vi "SetSize.vi"(9 "size":i32, 11 "PipeData in":refnum<class "StreamData.lvclass">) -> (3 "PipeData out":refnum<class "StreamData.lvclass">)   [LabVIEW 2017, in "Stream-t'WPI_EncoderType.ctl'.lvlib" / "StreamData.lvclass"]
uses:
  <extravilib>/ChannelInstances/Stream-t'WPI_EncoderType.ctl'/StreamData.lvclass
  <extravilib>/ChannelInstances/Stream-t'WPI_EncoderType.ctl'/StreamData.lvclass/StreamData.ctl
  <resource>/ChannelSupport/_ChannelSupport/PipeLogic/PipeLogic.lvclass/PipeLogic.ctl
  <resource>/ChannelSupport/_ChannelSupport/PipeLogic/PipeLogic.lvclass
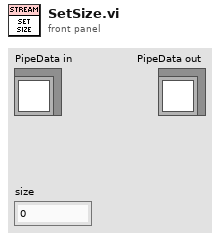
[diagram p1: front panel]
types:
  T1 = typedef "WPI_EncoderType.ctl" = enum16{"1x", "2x", "4x"}
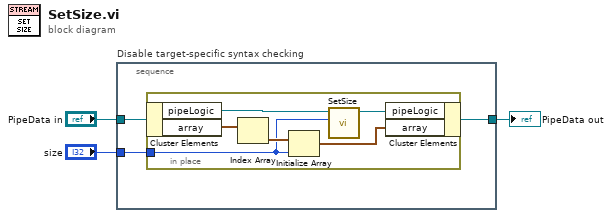
[diagram p0: block diagram]
diagram:
  n1 = stacked-sequence "Disable target-specific syntax checking" {
    tunnel: "PipeData in" -> [w6]
    tunnel: [w5] -> w2
    tunnel: "size" -> [w4]
    frame #0 {
      n2 = in-place {
        in-place-border: w4 -> [w7]
        n3 = in-place-cluster #1(w6) -> ("pipeLogic"=w9:refnum<class "PipeLogic.lvclass">, "array"=w12:cluster{"element":T1}[])
        n4 = Index Array(array=w12) -> (element=w11:cluster{"element":T1})  [unwired: 1 in]
        n5 = Initialize Array(w11, w7) -> (w10:cluster{"element":T1}[])
        n6 = call <resource>:"SetSize.vi"("size"=w7, "pipeLogic in"=w9) -> ("pipeLogic out"=w8:refnum<class "PipeLogic.lvclass">)  [unwired: 9 in]
        n7 = in-place-cluster #1("pipeLogic"=w8, "array"=w10) -> (w5:refnum<class "StreamData.lvclass">)
      }
    }
  }
  "PipeData out" <- w2
